vi "Read Route Enabled.vi"(8 "error in (no error)":errorcluster, 9 "Output Index":i32, 10 "Input Index":i32, 11 "VoiceMeeterRemote in":refnum<class "VoiceMeeterRemote.lvclass">) -> (0 "error out":errorcluster, 1 "Route Enabled?":bool, 2 "Parameter Name":string, 3 "VoiceMeeterRemote out":refnum<class "VoiceMeeterRemote.lvclass">)   [LabVIEW 2022 SP3, in "VoiceMeeterRemote.lvlib" / "VoiceMeeterRemote.lvclass"]
doc: "Returns whether audio is currently routed from the specified input index to the specified output index."
uses:
  VoiceMeeterRemote.lvclass
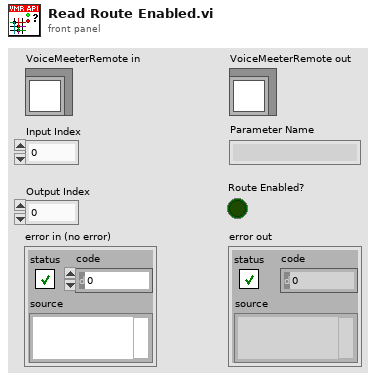
[diagram p1: front panel]
types:
  T1 = typedef "VoiceMeeterRemote.lvlib/Voicemeeter Type.ctl" = enum16{"Unknown", "Voicemeeter", "Banana", "Potato", "Potato x64"}
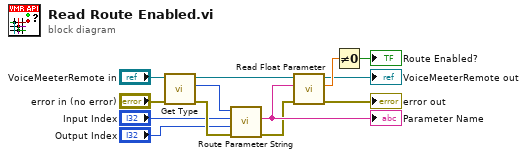
[diagram p0: block diagram]
diagram:
  n1 = call "Get Type.vi"("error in (no error)"="error in (no error)", "VoiceMeeterRemote in"="VoiceMeeterRemote in") -> ("error out"=w10:errorcluster, "Type"=w11:T1, "VoiceMeeterRemote out"=w7:refnum<class "VoiceMeeterRemote.lvclass">)  [unwired: 7 in]
  n2 = call "Route Parameter String.vi"("error in (no error)"=w10, "Output Index"="Output Index", "Input Index"="Input Index", "Voicemeeter Type"=w11) -> ("error out"=w5:errorcluster, "Route Parameter String"=w6:string)  [unwired: 6 in]
  "Parameter Name" <- w6
  n3 = call "Read Float Parameter.vi"("error in (no error)"=w5, "Parameter Name"=w6, "VoiceMeeterRemote in"=w7) -> ("error out"=→"error out":errorcluster, "Value"=w4:sgl, "VoiceMeeterRemote out"=→"VoiceMeeterRemote out":refnum<class "VoiceMeeterRemote.lvclass">)  [unwired: 6 in]
  n4 = Not Equal To 0?(x=w4) -> (x != 0?=→"Route Enabled?":bool)
